vi "TAT_PLC_TO_LabVIEW_Door_Status.vi"(7 "Enum":enum16{"Read", "Write"}(ring), 8 "error in (no error)":errorcluster, 10 "Array":bool[](array[boolean])) -> (0 "error out":errorcluster, 2 "Array 2":bool[](array[boolean]))   [LabVIEW 2017]
panel:
  # "DOOR OPEN CLOSE INPUT TO SOFT\t\nM461\tBACK 1\t8653\nM462\tBACK 2\t8654\nM463\tBACK 3\t8655\nM464\tBACK 4\t8656\nM465\tBACK 5\t8657\nM466\tBACK 6\t8658\nM467\tBACK 7\t8659\nM468\tBACK 8\t8660\nM469\tBACK 9\t8661\nM470\tBACK 10\t8662\nM471\tBACK 11\t8663\nM472\tFRONT 1\t8664\nM473\tFRONT 2\t8665\nM474\tFRONT 3\t8666\nM475\tFRONT 4\t8667\nM476\tFRONT 5\t8668\nM477\tFRONT 6\t8669\nM478\tFRONT 7\t8670\nM479\tFRONT 8\t8671\nM480\tFRONT 9\t8672\nM481\tFRONT 10\t8673\nM482\tFRONT 11\t8674\nM483\tBIN SEN 1\t8675\nM484\tBIN SEN 2\t8676\nM485\tBIN SEN 3\t8677\nM486\tBIN SEN 4\t8678\nM487\tBIN SEN 5\t8679"
  # "CONTROL PROCESS \n  PLC TO LabVIEW"
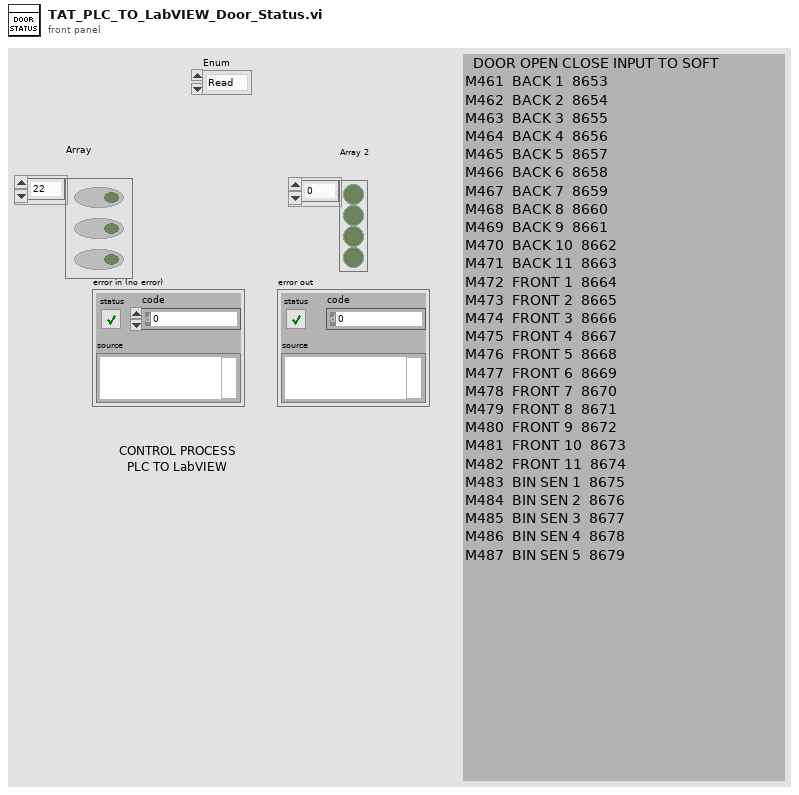
[diagram p1: front panel]
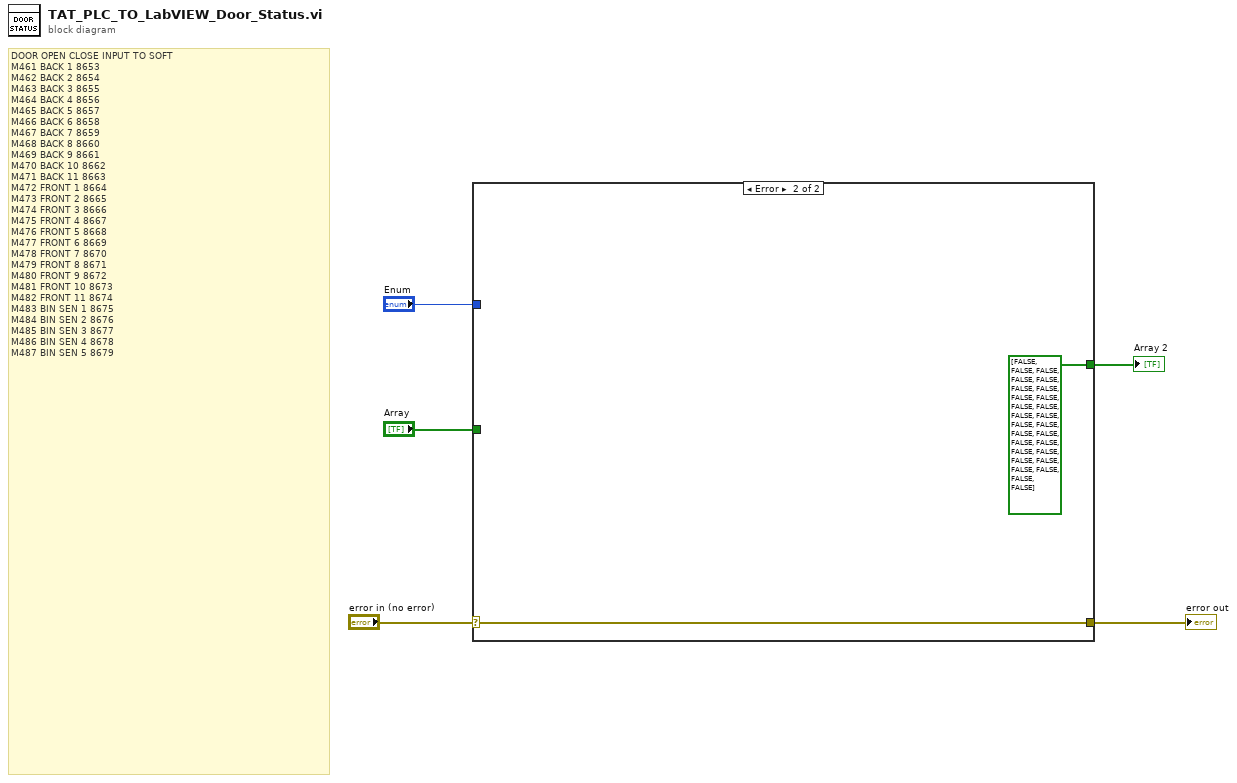
[diagram p0: block diagram]
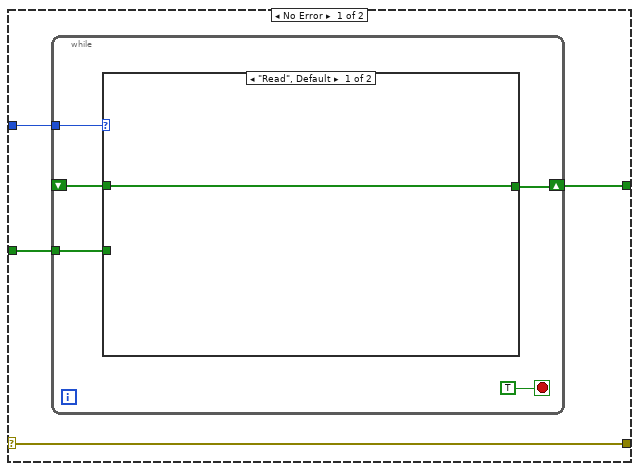
[diagram p2: hidden frame]
diagram:
  # "DOOR OPEN CLOSE INPUT TO SOFT\t\nM461\tBACK 1\t8653\nM462\tBACK 2\t8654\nM463\tBACK 3\t8655\nM464\tBACK 4\t8656\nM465\tBACK 5\t8657\nM466\tBACK 6\t8658\nM467\tBACK 7\t8659\nM468\tBACK 8\t8660\nM469\tBACK 9\t8661\nM470\tBACK 10\t8662\nM471\tBACK 11\t8663\nM472\tFRONT 1\t8664\nM473\tFRONT 2\t8665\nM474\tFRONT 3\t8666\nM475\tFRONT 4\t8667\nM476\tFRONT 5\t8668\nM477\tFRONT 6\t8669\nM478\tFRONT 7\t8670\nM479\tFRONT 8\t8671\nM480\tFRONT 9\t8672\nM481\tFRONT 10\t8673\nM482\tFRONT 11\t8674\nM483\tBIN SEN 1\t8675\nM484\tBIN SEN 2\t8676\nM485\tBIN SEN 3\t8677\nM486\tBIN SEN 4\t8678\nM487\tBIN SEN 5\t8679"
  n1 = case shown="Error" "error in (no error)" {
    selector: "error in (no error)" -> [w6 w18]
    tunnel: [w6 w18] -> w5
    tunnel: "Enum" -> [w9 _]
    tunnel: "Array" -> [w8 _]
    tunnel: [w7 bool[] [FALSE, FALSE, FALSE, FALSE, FALSE, FALSE, FALSE, FALSE, FALSE, FALSE, FALSE, FALSE, FALSE, FALSE, FALSE, FALSE, FALSE, FALSE, FALSE, FALSE, FALSE, FALSE, FALSE, FALSE, FALSE, FALSE, FALSE]] -> w1
    frame No Error {
      n2 = while {
        tunnel: w9 -> [w13]
        shift-right: [w10] -> w7
        shift-left: _ -> [w11]
        tunnel: w8 -> [w12]
        stop <- TRUE stop-if-true
        n3 = case shown="\"Read\", Default" w13 {
          tunnel: w12 -> [_ w16]
          tunnel: [w15 w16] -> w10
          tunnel: w11 -> [w15 _]
          frame "Read", Default {
          }
          frame "Write" {
          }
        }
      }
    }
    frame Error {
    }
  }
  "error out" <- w5
  "Array 2" <- w1
